vi "Test Verify CLI.vi"(11 "Test Case In":refnum<class "Core Library Error Propagation.lvclass">) -> (0 "error out":errorcluster, 3 "Test Case Out":refnum<class "Core Library Error Propagation.lvclass">)   [LabVIEW 2020, in "Core Library Error Propagation.lvclass"]
uses:
  Core Library Error Propagation.lvclass
  C:/Program Files/National Instruments/LabVIEW 2026/vi.lib/Astemes/LUnit/Test Case.lvclass
  Source/Approval Tests/Options/Options.lvclass
  Source/Approval Tests/Verify CLI Options.ctl
  <vilib>/Astemes/LUnit/Test Case.lvclass/Test Case.ctl
  <vilib>/Astemes/LUnit/Palette/Pass If Error.vi
  <vilib>/Astemes/LUnit/Palette/Advanced Assertions/Pass If Specific Error.vi/d0e67a5c-31db-4060-a993-98defbf94426.vi
  <vilib>/Astemes/LUnit/Palette/Fail.vi
  <vilib>/Astemes/LUnit/Core/LUnit Test Case/Private/Append Fail Result.vi
  <vilib>/Astemes/LUnit/Core/LUnit Test Case/Private/Append Pass Result.vi
  <vilib>/Astemes/LUnit/Core/LUnit Test Case/Private/Run In UI.vi
  <vilib>/Utility/error.llb/Clear Errors.vi
  <vilib>/Comparison/Equal/Equal Functor/Equal Functor.lvclass
  <vilib>/Astemes/LUnit/Palette/Advanced Assertions/LUnit Advanced Assertions.lvlib
  Source/Approval Tests/Approval Tests.lvlib
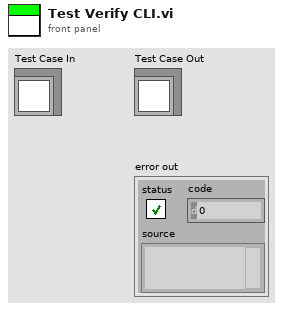
[diagram p1: front panel]
types:
  T1 = typedef "Approval Tests.lvlib/Verify CLI Options.ctl" = cluster{"standard input":string, "working directory":path, "expected output size  (4096)":u32, "Run Minimized (T)":bool}
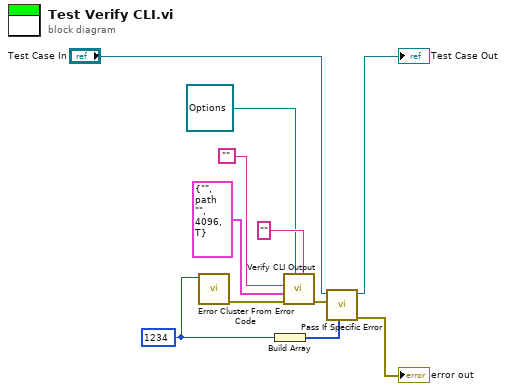
[diagram p0: block diagram]
diagram:
  w1 = 1234 ("error code (0)")
  n1 = call <vilib>:"Error Cluster From Error Code.vi"("error code (0)"=w1) -> ("error out"=w4:errorcluster)  [unwired: 8 in]
  n2 = Build Array(w1) -> (w3:i32[])
  n3 = call "Verify CLI Output.vi"("Label"="", "Approval Tests.lvlib:Options.lvclass"=refnum<class "Options.lvclass"> refnum, "error in"=w4, "CLI Options"=T1 {"standard input"="", "working directory"=path "", "expected output size  (4096)"=4096, "Run Minimized (T)"=TRUE}, "command line"="") -> ("error out"=w2:errorcluster)  [unwired: 4 in, 2 out]
  n4 = call <vilib>:"Pass If Specific Error.vi"("Error Codes"=w3, "Assert error"=w2, "LUnit Test Case In"="Test Case In") -> ("error out"=→"error out":errorcluster, "LUnit Test Case Out"=→"Test Case Out":refnum<class "Core Library Error Propagation.lvclass">)  [unwired: 7 in]
